vi "CIE-2 Tone.vi"(0 "AO Channels":i32[](array[numeric]), 1 "Ear":T2, 2 "Sampling Rate (Hz)":dbl=200000.0, 5 "Acoustic System":string, 7 "Probe mic gain (dB)":dbl, 9 "DP Freqs":T1, 11 "error in (no error)":errorcluster, 12 "Nominal Max SPLs":dbl[](array[numeric]), 13 "Override recal check?":bool) -> (4 "Max SPL1":dbl, 6 "Max SPL2":dbl, 15 "error out":errorcluster)   [LabVIEW 2020]
uses:
  epl-vi-lib/Utility VIs/Type Defs/Left-Right ring.ctl
  cfts/LV Source/DPOAE VIs/Typedefs/DP-Freqs.ctl
  epl-vi-lib/Utility VIs/Math VIs/FFTtoR,Theta (1D).VI
panel:
  in  "Averages":i32=2
  in  "Duration (s)":dbl=0.1
  out "Mag graph":dbl[](graph)
  out "Mic Signal":dbl[](graph)
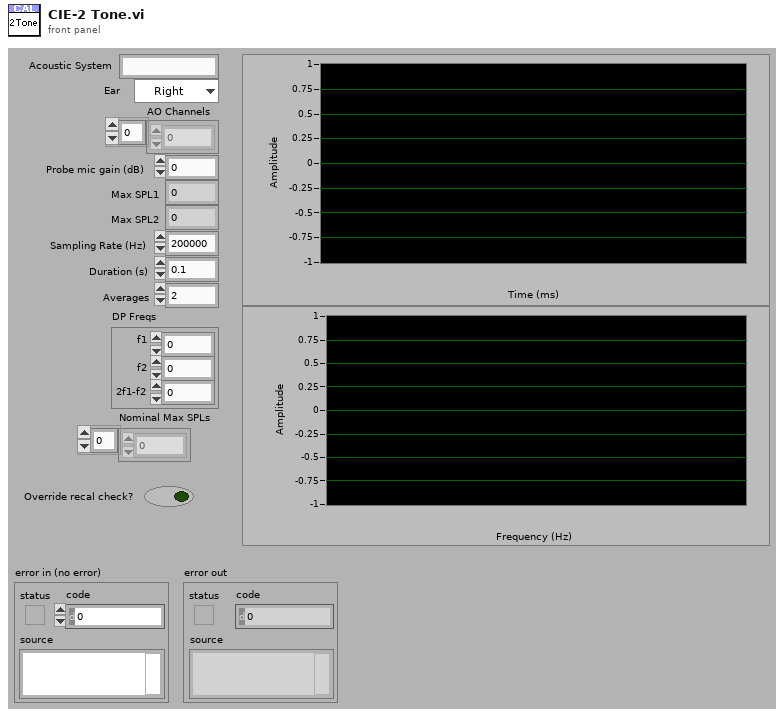
[diagram p1: front panel]
types:
  T1 = typedef "DP-Freqs.ctl" = cluster{"f1":dbl, "f2":dbl, "2f1-f2":dbl}
  T2 = typedef "Left-Right ring.ctl" = enum16{"Right", "Left"}
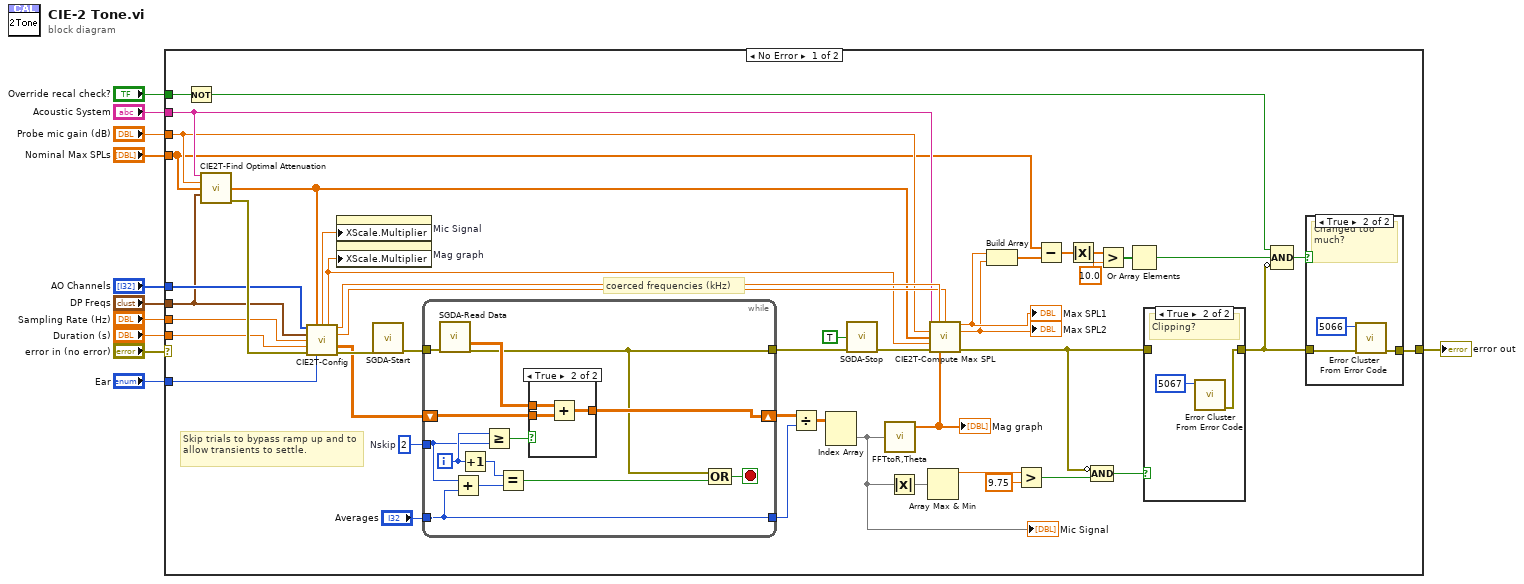
[diagram p0: block diagram]
diagram:
  n1 = case shown="No Error" "error in (no error)" {
    selector: "error in (no error)" -> [_ w82]
    tunnel: "Sampling Rate (Hz)" -> [w56 _]
    tunnel: "Duration (s)" -> [w55 _]
    tunnel: [w24 w82] -> w8
    tunnel: "DP Freqs" -> [w35 _]
    tunnel: "AO Channels" -> [w40 _]
    tunnel: "Acoustic System" -> [w39 _]
    tunnel: "Probe mic gain (dB)" -> [w37 _]
    tunnel: "Nominal Max SPLs" -> [w15 _]
    tunnel: "Ear" -> [w38 _]
    tunnel: "Override recal check?" -> [w14 _]
    frame No Error {
      w51 = 2  # Nskip
      # "coerced frequencies (kHz)"
      # "Skip trials to bypass ramp up and to allow transients to settle."
      n2 = Not(x=w14) -> (.not. x?=w13:bool)
      n3 = call "CIE2T-Find Optimal Attenuation.vi"("Acoustic System ID"=w39, "Probe mic gain (dB)"=w37, "Nominal Max SPL"=w15, "DP Freqs"=w35) -> ("Attenuation (dB)"=w32:dbl[], "error out"=w57:errorcluster)  [unwired: 10 in]
      n4 = call "CIE2T-Config.vi"("AO Channels"=w40, "Attenuation (dB)"=w32, "DP Freqs"=w35, "Sampling Rate (Hz)"=w56, "Duration (s)"=w55, "error in (no error)"=w57, "Ear"=w38) -> ("dt (ms)"=w47:dbl, "df (kHz)"=w36:dbl, "coerced f1 (kHz)"=w45:dbl, "coerced f2 (kHz)"=w43:dbl, "Mic Avg"=w44:dbl[][], "error out"=w54:errorcluster)  [unwired: 3 in]
      n5 = property on="Mic Signal" class="WFGraph (strict)"("XScale.Multiplier"=w47) -> ()  [unwired: 2 in, 2 out]
      n6 = property on="Mag graph" class="WFGraph (strict)"("XScale.Multiplier"=w36) -> ()  [unwired: 2 in, 2 out]
      n7 = call "SGDA-Start.vi"("error in (no error)"=w54) -> ("error out"=w53:errorcluster)  [unwired: 6 in]
      n8 = while {
        tunnel: w53 -> [w70]
        tunnel: [w58] -> w48
        tunnel: "Averages" -> [w59]
        shift-right: [w67] -> w50
        shift-left: w44 -> [w68]
        tunnel: w51 -> [w60]
        tunnel: [w59] -> w49
        i -> [w62]
        stop <- w66 stop-if-true
        n9 = call "SGDA-Read Data.vi"("error in (no error)"=w70) -> ("AI Waveforms"=w64:dbl[][], "error out"=w58:errorcluster)  [unwired: 13 in]
        n10 = Add(x=w60, y=w59) -> (x+y=w61:i32)
        n11 = Increment(x=w62) -> (x+1=w65:i32)
        n12 = Greater Or Equal?(x=w62, y=w60) -> (x >= y?=w63:bool)
        n13 = Equal?(x=w65, y=w61) -> (x = y?=w69:bool)
        n14 = case shown="True" w63 {
          tunnel: w68 -> [w71 w74]
          tunnel: [w71 w73] -> w67
          tunnel: w64 -> [_ w72]
          frame False {
          }
          frame True {
            n15 = Add(x=w72, y=w74) -> (x+y=w73:dbl[][])
          }
        }
        n16 = Compound Arithmetic op=OR(w58, w69) -> (w66:bool)
      }
      n17 = Divide(x=w50, y=w49) -> (x/y=w42:dbl[][])
      n18 = Index Array(array=w42) -> (element=w23:dbl[])  [unwired: 2 in]
      "Mic Signal" <- w23
      n19 = call "SGDA-Stop.vi"("Clear ActiveX (F)"=TRUE, "error in (no error)"=w48) -> ("error out"=w41:errorcluster)  [unwired: 13 in]
      n20 = call-poly "FFTtoR,Theta.VI"("X"=w23) -> ("+Freq. Mag of FFT"=w46:dbl[])  [unwired: 1 in, 1 out]
      "Mag graph" <- w46
      n21 = Absolute Value(x=w23) -> (abs(x)=w22:dbl[])
      n22 = Array Max & Min(array=w22) -> (max value=w21:dbl)  [unwired: 3 out]
      n23 = call "CIE2T-Compute Max SPL.vi"("Acoustic System"=w39, "f1 (kHz)"=w45, "f2 (kHz)"=w43, "Probe mic gain (dB)"=w37, "Attenuation (dB)"=w32, "df (kHz)"=w36, "error in (no error)"=w41, "+Freq. Mag of FFT"=w46) -> ("Max SPL1"=w34:dbl, "Max SPL2"=w33:dbl, "error out"=w18:errorcluster)  [unwired: 5 in]
      "Max SPL1" <- w34
      "Max SPL2" <- w33
      n24 = Build Array(w34, w33) -> (w31:dbl[])
      n25 = Greater?(x=w21, y=9.75) -> (0:w19:bool)
      n26 = Subtract(x=w15, y=w31) -> (x-y=w30:dbl[])
      n27 = Absolute Value(x=w30) -> (abs(x)=w29:dbl[])
      n28 = Compound Arithmetic op=AND(invert w18, w19) -> (w16:bool)
      n29 = Greater?(x=w29, y=10.0) -> (0:w27:bool[])
      n30 = Or Array Elements(Boolean array=w27) -> (logical OR=w26:bool)
      n31 = case shown="True" w16 {
        tunnel: w18 -> [w75 _]
        tunnel: [w75 w76] -> w17
        frame False {
        }
        frame True {
          # "Clipping?"
          n32 = call <vilib>:"Error Cluster From Error Code.vi"("error code (0)"=5067) -> ("error out"=w76:errorcluster)  [unwired: 8 in]
        }
      }
      n33 = Compound Arithmetic op=AND(w13, w26, invert w17) -> (w25:bool)
      n34 = case shown="True" w25 {
        tunnel: w17 -> [w78 w81]
        tunnel: [w78 w79] -> w24
        frame False {
        }
        frame True {
          # "Changed too much?"
          n35 = call <vilib>:"Error Cluster From Error Code.vi"("error in (no error)"=w81, "error code (0)"=5066) -> ("error out"=w79:errorcluster)  [unwired: 7 in]
        }
      }
    }
    frame Error {
    }
  }
  "error out" <- w8
